vi "initialize_params.vi"(1 "layer_nodes":i32[](array[numeric])) -> (0 "parameters":map{string, dbl[][]}(c390))   [LabVIEW 2020]
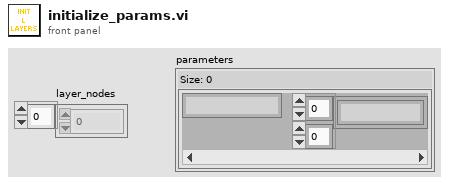
[diagram p1: front panel]
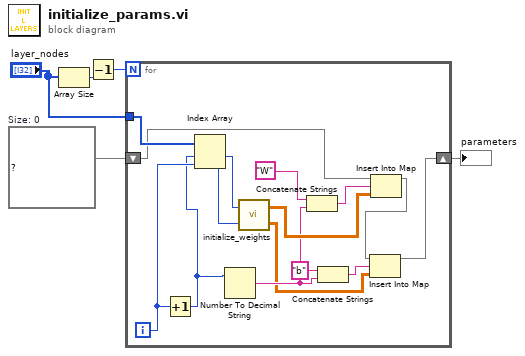
[diagram p0: block diagram]
diagram:
  w4 = map{string, dbl[][]} {}  # Size: 0
  n1 = Array Size(array="layer_nodes") -> (size(s)=w5:i32)
  n2 = Decrement(x=w5) -> (x-1=w1:i32)
  n3 = for {
    N: w1 -> [_]
    shift-right: [w6] -> w2
    shift-left: w4 -> [w12]
    tunnel: "layer_nodes" -> [w20]
    i -> [w19]
    n4 = Increment(x=w19) -> (x+1=w14:i32)
    n5 = Index Array(array=w20, index #1=w14, index #2=w19) -> (element #1=w18:i32, element #2=w17:i32)
    n6 = Number To Decimal String(number=w14) -> (decimal integer string=w10:string)  [unwired: 1 in]
    n7 = call "initialize_weights.vi"("n[l-1]"=w17, "n[l]"=w18) -> ("b"=w8:dbl[][], "W"=w13:dbl[][])
    n8 = Concatenate Strings("W", w10) -> (w16:string)
    n9 = Concatenate Strings("b" ("string"), w10) -> (w11:string)
    n10 = Insert Into Map(map in=w12, key=w16, value=w13) -> (map out=w7:map{string, dbl[][]})  [unwired: 2 out]
    n11 = Insert Into Map(map in=w7, key=w11, value=w8) -> (map out=w6:map{string, dbl[][]})  [unwired: 2 out]
  }
  "parameters" <- w2
